vi "OSQ_save.vi"(8 "error in (no error)":errorcluster, 10 "SEQs":T1[](array[typedef]), 11 "Save":path=path "C:/Users/Adam/Desktop/test.osq") -> (0 "error out":errorcluster, 3 "XML File Path(duplicate)":path)   [LabVIEW 2013]
uses:
  Line.ctl
  <vilib>/Utility/xml.llb/Write to XML File(string).vi
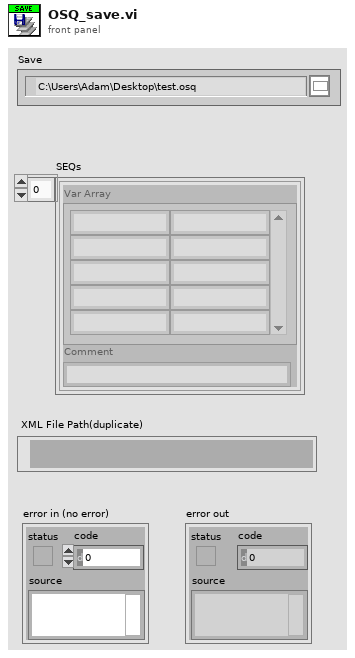
[diagram p1: front panel]
types:
  T1 = typedef "Line.ctl" = cluster{"Var Array":string[][], "Comment":string}
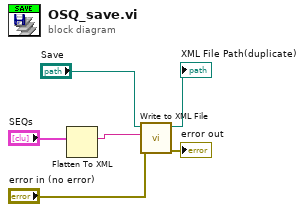
[diagram p0: block diagram]
diagram:
  n1 = Flatten To XML(anything="SEQs") -> (xml string=w5:string)
  n2 = call-poly <vilib>:"Write to XML File.vi"("error in (no error)"="error in (no error)", "XML Input"=w5, "XML File Path"="Save") -> ("error out"=→"error out":errorcluster, "XML File Path(duplicate)"=→"XML File Path(duplicate)":path)  [unwired: 6 in, 1 out]
